vi "Read Buffer.vi"(8 "error in (no error)":errorcluster, 10 "buffer in":u8[](array[numeric]), 11 "Buffer data":T1={"Buffer"=refnum, "Status"=refnum, "decimation"=0, "avg bandwidth"=0.0, "data type"=enum."Bool", "units"="", "channels"=[], "channel"=FALSE, "engine (T) / string (F)"=FALSE, "byte order"=enum."little-endian"} {"channels"."string offset" format="%d bytes"; "avg bandwidth" format="%.0g bytes"}) -> (0 "error out":errorcluster, 2 "buffer out":u8[](array[numeric]), 3 "buffer string":string, 5 "buffer size":u64, 7 "null?":bool)   [LabVIEW 2017, in "DSF Core.lvlib"]
uses:
  DSF Core.lvlib
  Buffer Data.ctl
  Classes/Buffer/Buffer.lvclass
  C:/Git/DSF/LabVIEW-Memory/Source/Classes/Pointer/Pointer.lvclass
  Classes/Transfer Group Status/Status.lvclass
  Typedefs/DSF Data Type.ctl
  Typedefs/DSF Engine Channel Configuration.ctl
  Typedefs/DSF Settings Info.ctl
  Typedefs/DSF Byte Order.ctl
  LabVIEW-Memory/Source/Classes/Pointer/Get Size.vi
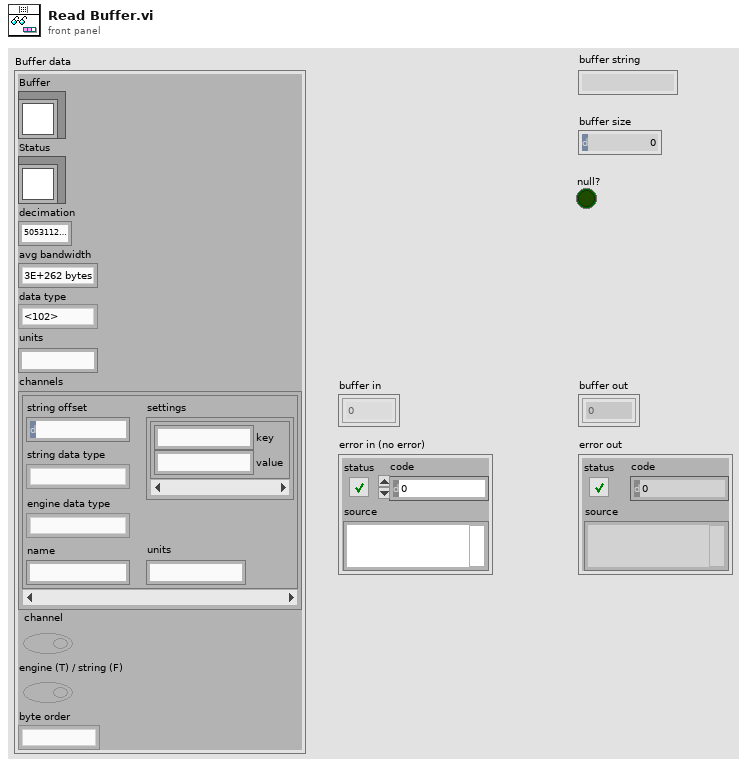
[diagram p1: front panel]
types:
  T1 = typedef "DSF Core.lvlib/Buffer Data.ctl" = cluster{"Buffer":refnum<class "Buffer.lvclass">, "Status":refnum<class "Status.lvclass">, "decimation":u64, "avg bandwidth":dbl, "data type":T2, "units":string, "channels":T3[], "channel":bool, "engine (T) / string (F)":bool, "byte order":T5}
  T2 = typedef "DSF Core.lvlib/DSF Data Type.ctl" = enum8{"Bool", "SGL", "DBL", "I8", "I16", "I32", "I64", "U8", "U16", "U32", "U64"}
  T3 = typedef "DSF Core.lvlib/DSF Engine Channel Configuration.ctl" = cluster{"string offset":u64, "string data type":T2, "engine data type":T2, "name":string, "settings":T4, "units":string}
  T4 = typedef "DSF Core.lvlib/DSF Settings Info.ctl" = cluster{"key":string, "value":string}[]
  T5 = typedef "DSF Core.lvlib/DSF Byte Order.ctl" = enum8{"big-endian", "little-endian"}
  T6 = enum16{"big-endian, network order", "native, host order", "little-endian"}
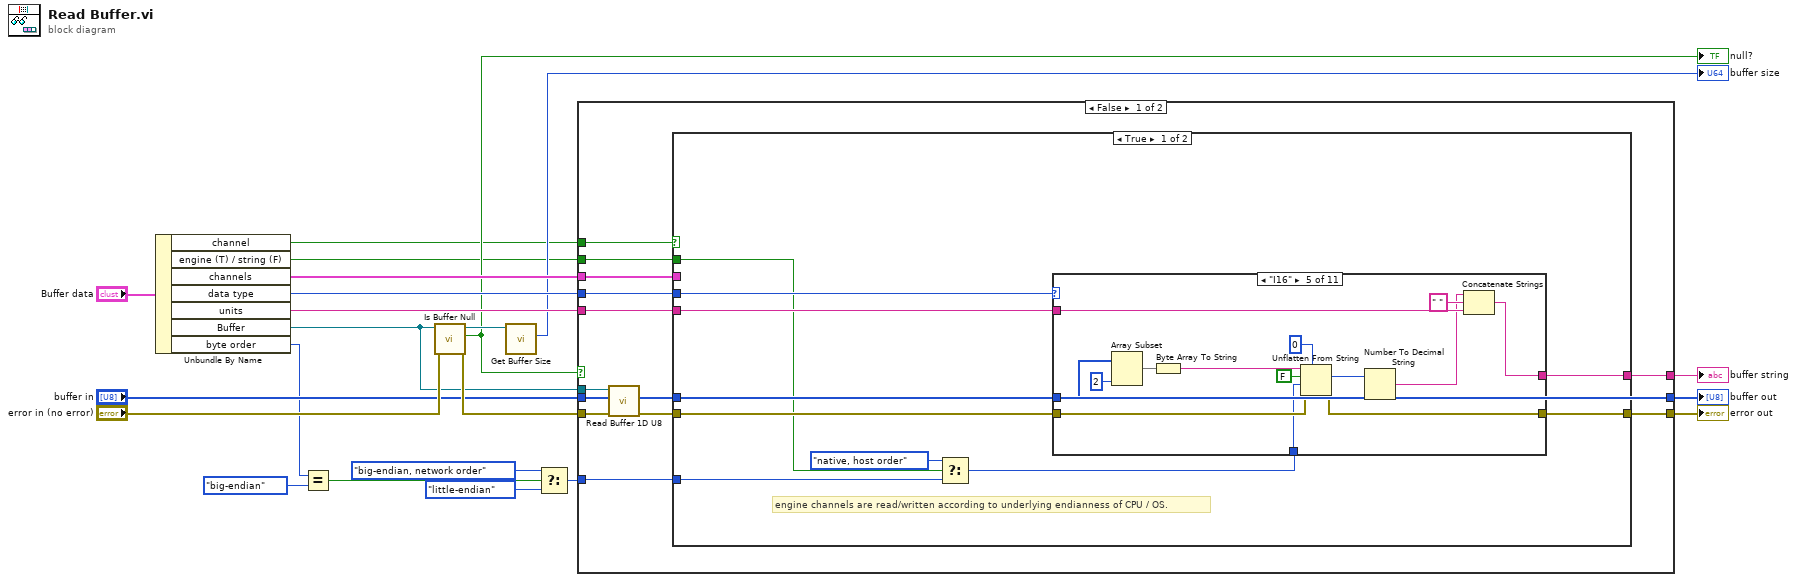
[diagram p0: block diagram]
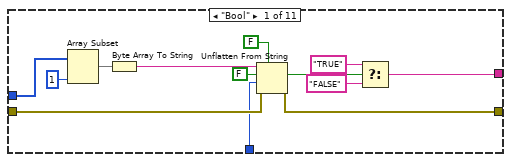
[diagram p2: hidden frame]
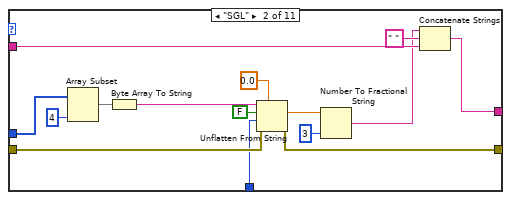
[diagram p3: hidden frame]
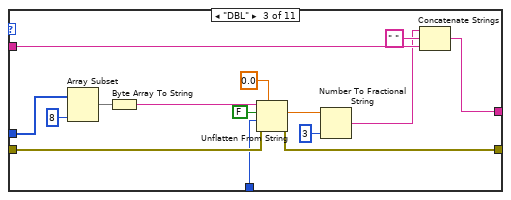
[diagram p4: hidden frame]
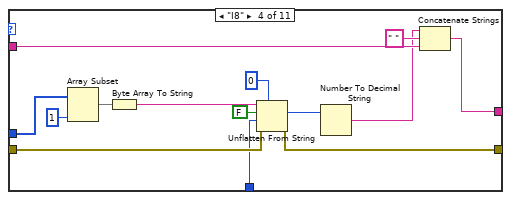
[diagram p5: hidden frame]
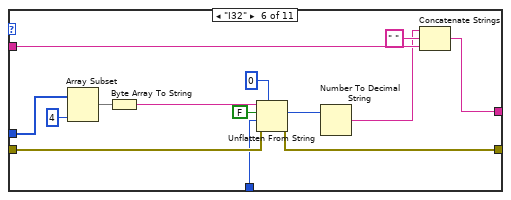
[diagram p6: hidden frame]
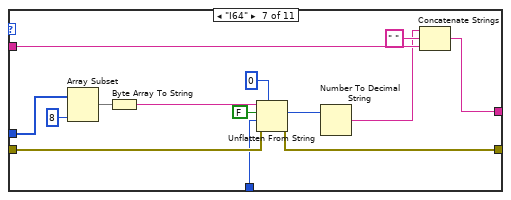
[diagram p7: hidden frame]
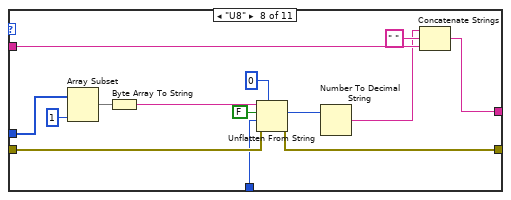
[diagram p8: hidden frame]
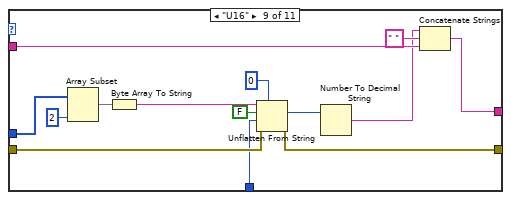
[diagram p9: hidden frame]
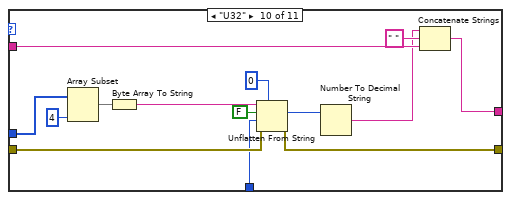
[diagram p10: hidden frame]
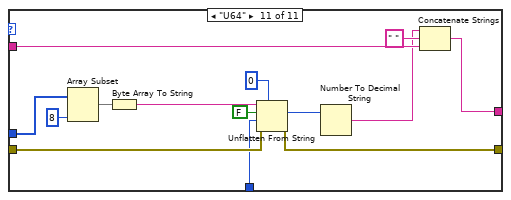
[diagram p11: hidden frame]
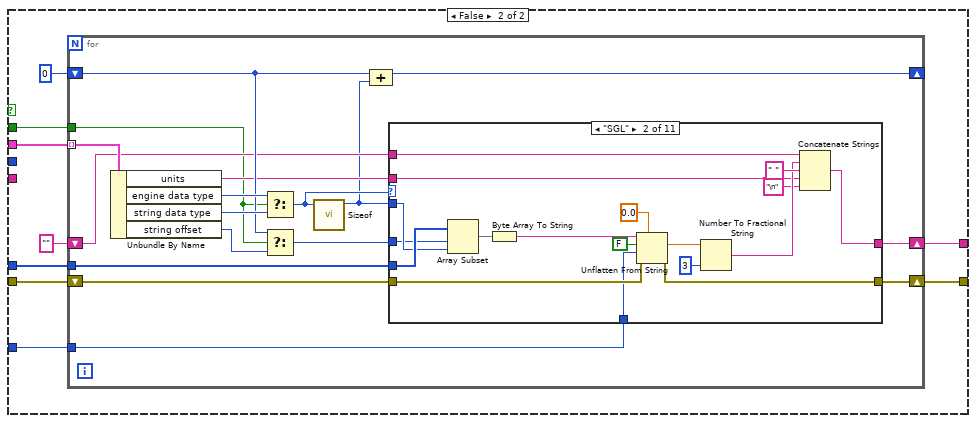
[diagram p12: hidden frame]
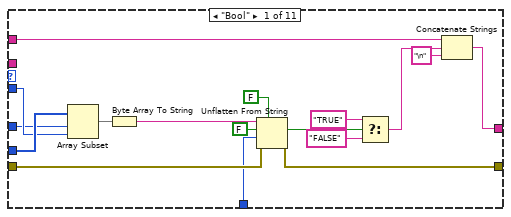
[diagram p13: hidden frame]
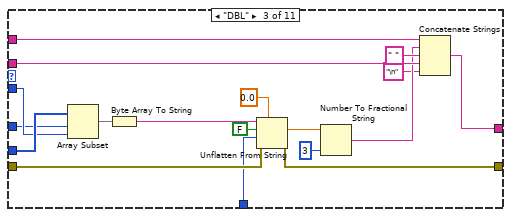
[diagram p14: hidden frame]
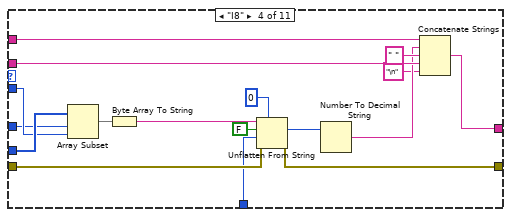
[diagram p15: hidden frame]
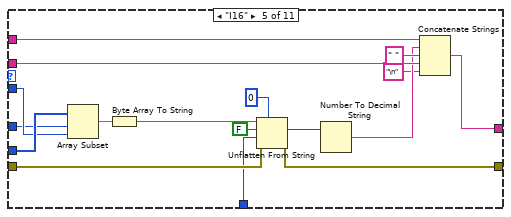
[diagram p16: hidden frame]
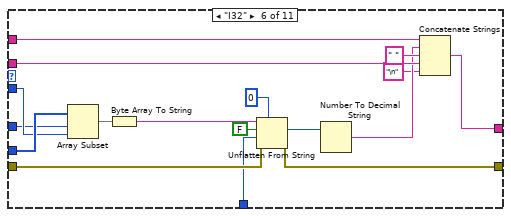
[diagram p17: hidden frame]
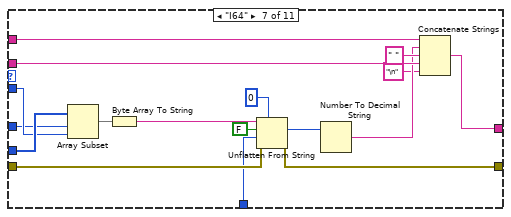
[diagram p18: hidden frame]
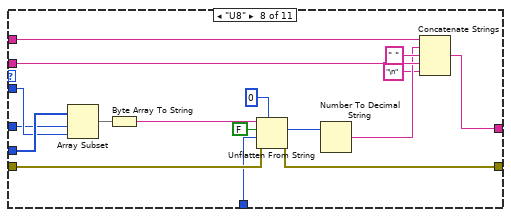
[diagram p19: hidden frame]
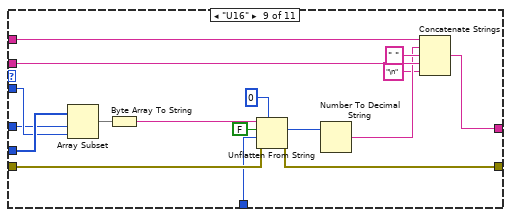
[diagram p20: hidden frame]
diagram:
  n1 = Unbundle By Name("Buffer data") -> ("channel"=w8:bool, "engine (T) / string (F)"=w7:bool, "channels"=w12:T3[], "data type"=w20:T2, "units"=w19:string, "Buffer"=w17:refnum<class "Buffer.lvclass">, "byte order"=w4:T5)
  n2 = Equal?(x=w4, y=DSF_Byte_Order."big-endian") -> (x = y?=w6:bool)
  n3 = call "Is Buffer Null.vi"("error in (no error)"="error in (no error)", "Buffer in"=w17) -> ("error out"=w18:errorcluster, "null?"=w10:bool, "Buffer out"=w22:refnum<class "Buffer.lvclass">)  [unwired: 7 in]
  "null?" <- w10
  n4 = call "Get Buffer Size.vi"("Buffer in"=w22) -> ("buffer size"=→"buffer size":u64)  [unwired: 9 in, 1 out]
  n5 = Select(t=T6."big-endian, network order" ("byte order (0:big-endian, network order)"), s=w6, f=T6."little-endian") -> (s? t:f=w1:T6)
  n6 = case shown="False" w10 {
    tunnel: w20 -> [w35 _]
    tunnel: w19 -> [w24 _]
    tunnel: w18 -> [w34 w416]
    tunnel: w17 -> [w33 _]
    tunnel: "buffer in" -> [w32 w418]
    tunnel: [w30 w416] -> w15
    tunnel: [w29 w418] -> w14
    tunnel: [w28 ""] -> w13
    tunnel: w8 -> [w27 _]
    tunnel: w12 -> [w26 _]
    tunnel: w7 -> [w25 _]
    tunnel: w1 -> [w23 _]
    frame False {
      n7 = call "Read Buffer 1D U8.vi"("error in (no error)"=w34, "dst array in"=w32, "Buffer in"=w33) -> ("error out"=w31:errorcluster, "dst array out"=w29:u8[])  [unwired: 5 in, 2 out]
      n8 = case shown="True" w27 {
        tunnel: w35 -> [w45 _]
        tunnel: w24 -> [w44 _]
        tunnel: w31 -> [w43 w209]
        tunnel: [w42 w208] -> w30
        tunnel: w29 -> [w41 w207]
        tunnel: [w40 w204] -> w28
        tunnel: w26 -> [_ w206]
        tunnel: w25 -> [w39 w205]
        tunnel: w23 -> [w37 w201]
        frame True {
          # "engine channels are read/written according to underlying endianness of CPU / OS."
          n9 = Select(t=T6."native, host order", s=w39, f=w37) -> (s? t:f=w36:T6)
          n10 = case shown="\"I16\"" w45 {
            tunnel: w41 -> [w58 w73 w88 w102 w116 w130 w144 w158 w172 w186 w200]
            tunnel: w44 -> [_ w62 w77 w92 w106 w120 w134 w148 w162 w176 w190]
            tunnel: w43 -> [w55 w70 w85 w99 w113 w127 w141 w155 w169 w183 w197]
            tunnel: [w54 w69 w84 w98 w112 w126 w140 w154 w168 w182 w196] -> w42
            tunnel: [w47 w61 w76 w91 w105 w119 w133 w147 w161 w175 w189] -> w40
            tunnel: w36 -> [w46 w59 w74 w89 w103 w117 w131 w145 w159 w173 w187]
            frame "Bool" {
              n11 = Array Subset(array=w58, length=1) -> (w56:u8[])  [unwired: 1 in]
              n12 = Byte Array To String(unsigned byte array=w56) -> (string=w53:string)
              n13 = Unflatten From String(type=FALSE, binary string=w53, data includes array or string size? (T)=FALSE, byte order (0:big-endian, network order)=w46, error in (no error)=w55) -> (value=w50:bool, error out=w54:errorcluster)  [unwired: 1 out]
              n14 = Select(t="TRUE", s=w50, f="FALSE") -> (s? t:f=w47:string)
            }
            frame "SGL" {
              n15 = Array Subset(array=w73, length=4) -> (w71:u8[])  [unwired: 1 in]
              n16 = Byte Array To String(unsigned byte array=w71) -> (string=w68:string)
              n17 = Unflatten From String(type=sgl 0.0, binary string=w68, data includes array or string size? (T)=FALSE, byte order (0:big-endian, network order)=w59, error in (no error)=w70) -> (value=w65:sgl, error out=w69:errorcluster)  [unwired: 1 out]
              n18 = Number To Fractional String(number=w65, precision (6)=i16 3) -> (F-format string=w60:string)  [unwired: 2 in]
              n19 = Concatenate Strings(w60, " " ("string"), w62) -> (w61:string)
            }
            frame "DBL" {
              n20 = Array Subset(array=w88, length=8) -> (w86:u8[])  [unwired: 1 in]
              n21 = Byte Array To String(unsigned byte array=w86) -> (string=w83:string)
              n22 = Unflatten From String(type=0.0, binary string=w83, data includes array or string size? (T)=FALSE, byte order (0:big-endian, network order)=w74, error in (no error)=w85) -> (value=w80:dbl, error out=w84:errorcluster)  [unwired: 1 out]
              n23 = Number To Fractional String(number=w80, precision (6)=i16 3) -> (F-format string=w75:string)  [unwired: 2 in]
              n24 = Concatenate Strings(w75, " " ("string"), w77) -> (w76:string)
            }
            frame "I8" {
              n25 = Array Subset(array=w102, length=1) -> (w100:u8[])  [unwired: 1 in]
              n26 = Byte Array To String(unsigned byte array=w100) -> (string=w97:string)
              n27 = Unflatten From String(type=i8 0, binary string=w97, data includes array or string size? (T)=FALSE, byte order (0:big-endian, network order)=w89, error in (no error)=w99) -> (value=w94:i8, error out=w98:errorcluster)  [unwired: 1 out]
              n28 = Number To Decimal String(number=w94) -> (decimal integer string=w90:string)  [unwired: 1 in]
              n29 = Concatenate Strings(w90, " " ("string"), w92) -> (w91:string)
            }
            frame "I16" {
              n30 = Array Subset(array=w116, length=2) -> (w114:u8[])  [unwired: 1 in]
              n31 = Byte Array To String(unsigned byte array=w114) -> (string=w111:string)
              n32 = Unflatten From String(type=i16 0, binary string=w111, data includes array or string size? (T)=FALSE, byte order (0:big-endian, network order)=w103, error in (no error)=w113) -> (value=w108:i16, error out=w112:errorcluster)  [unwired: 1 out]
              n33 = Number To Decimal String(number=w108) -> (decimal integer string=w104:string)  [unwired: 1 in]
              n34 = Concatenate Strings(w104, " " ("string"), w106) -> (w105:string)
            }
            frame "I32" {
              n35 = Array Subset(array=w130, length=4) -> (w128:u8[])  [unwired: 1 in]
              n36 = Byte Array To String(unsigned byte array=w128) -> (string=w125:string)
              n37 = Unflatten From String(type=0, binary string=w125, data includes array or string size? (T)=FALSE, byte order (0:big-endian, network order)=w117, error in (no error)=w127) -> (value=w122:i32, error out=w126:errorcluster)  [unwired: 1 out]
              n38 = Number To Decimal String(number=w122) -> (decimal integer string=w118:string)  [unwired: 1 in]
              n39 = Concatenate Strings(w118, " " ("string"), w120) -> (w119:string)
            }
            frame "I64" {
              n40 = Array Subset(array=w144, length=8) -> (w142:u8[])  [unwired: 1 in]
              n41 = Byte Array To String(unsigned byte array=w142) -> (string=w139:string)
              n42 = Unflatten From String(type=i64 0, binary string=w139, data includes array or string size? (T)=FALSE, byte order (0:big-endian, network order)=w131, error in (no error)=w141) -> (value=w136:i64, error out=w140:errorcluster)  [unwired: 1 out]
              n43 = Number To Decimal String(number=w136) -> (decimal integer string=w132:string)  [unwired: 1 in]
              n44 = Concatenate Strings(w132, " " ("string"), w134) -> (w133:string)
            }
            frame "U8" {
              n45 = Array Subset(array=w158, length=1) -> (w156:u8[])  [unwired: 1 in]
              n46 = Byte Array To String(unsigned byte array=w156) -> (string=w153:string)
              n47 = Unflatten From String(type=u8 0, binary string=w153, data includes array or string size? (T)=FALSE, byte order (0:big-endian, network order)=w145, error in (no error)=w155) -> (value=w150:u8, error out=w154:errorcluster)  [unwired: 1 out]
              n48 = Number To Decimal String(number=w150) -> (decimal integer string=w146:string)  [unwired: 1 in]
              n49 = Concatenate Strings(w146, " " ("string"), w148) -> (w147:string)
            }
            frame "U16" {
              n50 = Array Subset(array=w172, length=2) -> (w170:u8[])  [unwired: 1 in]
              n51 = Byte Array To String(unsigned byte array=w170) -> (string=w167:string)
              n52 = Unflatten From String(type=u16 0, binary string=w167, data includes array or string size? (T)=FALSE, byte order (0:big-endian, network order)=w159, error in (no error)=w169) -> (value=w164:u16, error out=w168:errorcluster)  [unwired: 1 out]
              n53 = Number To Decimal String(number=w164) -> (decimal integer string=w160:string)  [unwired: 1 in]
              n54 = Concatenate Strings(w160, " " ("string"), w162) -> (w161:string)
            }
            frame "U32" {
              n55 = Array Subset(array=w186, length=4) -> (w184:u8[])  [unwired: 1 in]
              n56 = Byte Array To String(unsigned byte array=w184) -> (string=w181:string)
              n57 = Unflatten From String(type=u32 0, binary string=w181, data includes array or string size? (T)=FALSE, byte order (0:big-endian, network order)=w173, error in (no error)=w183) -> (value=w178:u32, error out=w182:errorcluster)  [unwired: 1 out]
              n58 = Number To Decimal String(number=w178) -> (decimal integer string=w174:string)  [unwired: 1 in]
              n59 = Concatenate Strings(w174, " " ("string"), w176) -> (w175:string)
            }
            frame "U64" {
              n60 = Array Subset(array=w200, length=8) -> (w198:u8[])  [unwired: 1 in]
              n61 = Byte Array To String(unsigned byte array=w198) -> (string=w195:string)
              n62 = Unflatten From String(type=u64 0, binary string=w195, data includes array or string size? (T)=FALSE, byte order (0:big-endian, network order)=w187, error in (no error)=w197) -> (value=w192:u64, error out=w196:errorcluster)  [unwired: 1 out]
              n63 = Number To Decimal String(number=w192) -> (decimal integer string=w188:string)  [unwired: 1 in]
              n64 = Concatenate Strings(w188, " " ("string"), w190) -> (w189:string)
            }
          }
        }
        frame False {
          n65 = for {
            tunnel: w207 -> [w224]
            shift-right: [w225] -> w208
            shift-left: w209 -> [w226]
            tunnel: w206 -> [w223] mode=indexing
            tunnel: w205 -> [w211]
            shift-right: [w216] -> w204
            shift-left: "" -> [w214]
            shift-right: [w217] -> _
            shift-left: u64 0 -> [w218]
            tunnel: w201 -> [w210]
            n66 = Unbundle By Name(w223) -> ("units"=w215:string, "engine data type"=w219:T2, "string data type"=w220:T2, "string offset"=w222:u64)
            n67 = Select(t=w219, s=w211, f=w220) -> (s? t:f=w213:T2)
            n68 = Select(t=w218, s=w211, f=w222) -> (s? t:f=w221:u64)
            n69 = call "Sizeof.vi"("data type"=w213) -> ("size in bytes"=w212:u64)  [unwired: 9 in, 1 out]
            n70 = Compound Arithmetic op=ADD(w218, w212) -> (w217:u64)
            n71 = case shown="\"SGL\"" w213 {
              tunnel: w224 -> [w243 w261 w279 w296 w313 w330 w347 w364 w381 w398 w415]
              tunnel: w215 -> [_ w247 w269 w287 w304 w321 w338 w355 w373 w389 w406]
              tunnel: w226 -> [w241 w259 w277 w294 w311 w328 w345 w362 w379 w396 w413]
              tunnel: [w240 w258 w276 w293 w310 w327 w344 w361 w365 w395 w412] -> w225
              tunnel: [w231 w251 w268 w286 w303 w320 w337 w354 w372 w388 w405] -> w216
              tunnel: w221 -> [w228 w245 w263 w281 w298 w315 w332 w349 w367 w383 w403]
              tunnel: w212 -> [w229 w246 w264 w282 w299 w316 w333 w350 w368 w384 w400]
              tunnel: w214 -> [w233 w249 w266 w284 w301 w318 w335 w352 w370 w386 w402]
              tunnel: w210 -> [w227 w244 w262 w280 w297 w314 w331 w348 w366 w382 w399]
              frame "Bool" {
                n72 = Array Subset(array=w243, index=w228, length=w229) -> (w242:u8[])
                n73 = Byte Array To String(unsigned byte array=w242) -> (string=w239:string)
                n74 = Unflatten From String(type=FALSE, binary string=w239, data includes array or string size? (T)=FALSE, byte order (0:big-endian, network order)=w227, error in (no error)=w241) -> (value=w236:bool, error out=w240:errorcluster)  [unwired: 1 out]
                n75 = Select(t="TRUE", s=w236, f="FALSE") -> (s? t:f=w232:string)
                n76 = Concatenate Strings(w233, w232, "\n" ("string")) -> (w231:string)
              }
              frame "SGL" {
                n77 = Array Subset(array=w261, index=w245, length=w246) -> (w260:u8[])
                n78 = Byte Array To String(unsigned byte array=w260) -> (string=w257:string)
                n79 = Unflatten From String(type=sgl 0.0, binary string=w257, data includes array or string size? (T)=FALSE, byte order (0:big-endian, network order)=w244, error in (no error)=w259) -> (value=w254:sgl, error out=w258:errorcluster)  [unwired: 1 out]
                n80 = Number To Fractional String(number=w254, precision (6)=i16 3) -> (F-format string=w250:string)  [unwired: 2 in]
                n81 = Concatenate Strings(w249, w250, " " ("string"), w247, "\n" ("string")) -> (w251:string)
              }
              frame "DBL" {
                n82 = Array Subset(array=w279, index=w263, length=w264) -> (w278:u8[])
                n83 = Byte Array To String(unsigned byte array=w278) -> (string=w275:string)
                n84 = Unflatten From String(type=0.0, binary string=w275, data includes array or string size? (T)=FALSE, byte order (0:big-endian, network order)=w262, error in (no error)=w277) -> (value=w272:dbl, error out=w276:errorcluster)  [unwired: 1 out]
                n85 = Number To Fractional String(number=w272, precision (6)=i16 3) -> (F-format string=w267:string)  [unwired: 2 in]
                n86 = Concatenate Strings(w266, w267, " " ("string"), w269, "\n" ("string")) -> (w268:string)
              }
              frame "I8" {
                n87 = Array Subset(array=w296, index=w281, length=w282) -> (w295:u8[])
                n88 = Byte Array To String(unsigned byte array=w295) -> (string=w292:string)
                n89 = Unflatten From String(type=i8 0, binary string=w292, data includes array or string size? (T)=FALSE, byte order (0:big-endian, network order)=w280, error in (no error)=w294) -> (value=w289:i8, error out=w293:errorcluster)  [unwired: 1 out]
                n90 = Number To Decimal String(number=w289) -> (decimal integer string=w285:string)  [unwired: 1 in]
                n91 = Concatenate Strings(w284, w285, " " ("string"), w287, "\n" ("string")) -> (w286:string)
              }
              frame "I16" {
                n92 = Array Subset(array=w313, index=w298, length=w299) -> (w312:u8[])
                n93 = Byte Array To String(unsigned byte array=w312) -> (string=w309:string)
                n94 = Unflatten From String(type=i16 0, binary string=w309, data includes array or string size? (T)=FALSE, byte order (0:big-endian, network order)=w297, error in (no error)=w311) -> (value=w306:i16, error out=w310:errorcluster)  [unwired: 1 out]
                n95 = Number To Decimal String(number=w306) -> (decimal integer string=w302:string)  [unwired: 1 in]
                n96 = Concatenate Strings(w301, w302, " " ("string"), w304, "\n" ("string")) -> (w303:string)
              }
              frame "I32" {
                n97 = Array Subset(array=w330, index=w315, length=w316) -> (w329:u8[])
                n98 = Byte Array To String(unsigned byte array=w329) -> (string=w326:string)
                n99 = Unflatten From String(type=0, binary string=w326, data includes array or string size? (T)=FALSE, byte order (0:big-endian, network order)=w314, error in (no error)=w328) -> (value=w323:i32, error out=w327:errorcluster)  [unwired: 1 out]
                n100 = Number To Decimal String(number=w323) -> (decimal integer string=w319:string)  [unwired: 1 in]
                n101 = Concatenate Strings(w318, w319, " " ("string"), w321, "\n" ("string")) -> (w320:string)
              }
              frame "I64" {
                n102 = Array Subset(array=w347, index=w332, length=w333) -> (w346:u8[])
                n103 = Byte Array To String(unsigned byte array=w346) -> (string=w343:string)
                n104 = Unflatten From String(type=i64 0, binary string=w343, data includes array or string size? (T)=FALSE, byte order (0:big-endian, network order)=w331, error in (no error)=w345) -> (value=w340:i64, error out=w344:errorcluster)  [unwired: 1 out]
                n105 = Number To Decimal String(number=w340) -> (decimal integer string=w336:string)  [unwired: 1 in]
                n106 = Concatenate Strings(w335, w336, " " ("string"), w338, "\n" ("string")) -> (w337:string)
              }
              frame "U8" {
                n107 = Array Subset(array=w364, index=w349, length=w350) -> (w363:u8[])
                n108 = Byte Array To String(unsigned byte array=w363) -> (string=w360:string)
                n109 = Unflatten From String(type=u8 0, binary string=w360, data includes array or string size? (T)=FALSE, byte order (0:big-endian, network order)=w348, error in (no error)=w362) -> (value=w357:u8, error out=w361:errorcluster)  [unwired: 1 out]
                n110 = Number To Decimal String(number=w357) -> (decimal integer string=w353:string)  [unwired: 1 in]
                n111 = Concatenate Strings(w352, w353, " " ("string"), w355, "\n" ("string")) -> (w354:string)
              }
              frame "U16" {
                n112 = Array Subset(array=w381, index=w367, length=w368) -> (w380:u8[])
                n113 = Byte Array To String(unsigned byte array=w380) -> (string=w378:string)
                n114 = Unflatten From String(type=u16 0, binary string=w378, data includes array or string size? (T)=FALSE, byte order (0:big-endian, network order)=w366, error in (no error)=w379) -> (value=w375:u16, error out=w365:errorcluster)  [unwired: 1 out]
                n115 = Number To Decimal String(number=w375) -> (decimal integer string=w371:string)  [unwired: 1 in]
                n116 = Concatenate Strings(w370, w371, " " ("string"), w373, "\n" ("string")) -> (w372:string)
              }
              frame "U32" {
                n117 = Array Subset(array=w398, index=w383, length=w384) -> (w397:u8[])
                n118 = Byte Array To String(unsigned byte array=w397) -> (string=w394:string)
                n119 = Unflatten From String(type=u32 0, binary string=w394, data includes array or string size? (T)=FALSE, byte order (0:big-endian, network order)=w382, error in (no error)=w396) -> (value=w391:u32, error out=w395:errorcluster)  [unwired: 1 out]
                n120 = Number To Decimal String(number=w391) -> (decimal integer string=w387:string)  [unwired: 1 in]
                n121 = Concatenate Strings(w386, w387, " " ("string"), w389, "\n" ("string")) -> (w388:string)
              }
              frame "U64" {
                n122 = Array Subset(array=w415, index=w403, length=w400) -> (w414:u8[])
                n123 = Byte Array To String(unsigned byte array=w414) -> (string=w411:string)
                n124 = Unflatten From String(type=u64 0, binary string=w411, data includes array or string size? (T)=FALSE, byte order (0:big-endian, network order)=w399, error in (no error)=w413) -> (value=w408:u64, error out=w412:errorcluster)  [unwired: 1 out]
                n125 = Number To Decimal String(number=w408) -> (decimal integer string=w404:string)  [unwired: 1 in]
                n126 = Concatenate Strings(w402, w404, " " ("string"), w406, "\n" ("string")) -> (w405:string)
              }
            }
          }
        }
      }
    }
    frame True {
    }
  }
  "error out" <- w15
  "buffer out" <- w14
  "buffer string" <- w13
